vi "Frequency to phase word DBL.vi"(9 "Phase word base":i64=4294967296 format="0x%x (%d)", 10 "DDS clock":dbl=125000000.0 format="%_13p", 11 "Frequency":dbl format="%#_15p") -> (3 "Phase word":u64=1717987 format="0x%x (%d) 0b%b")   [LabVIEW 2015]
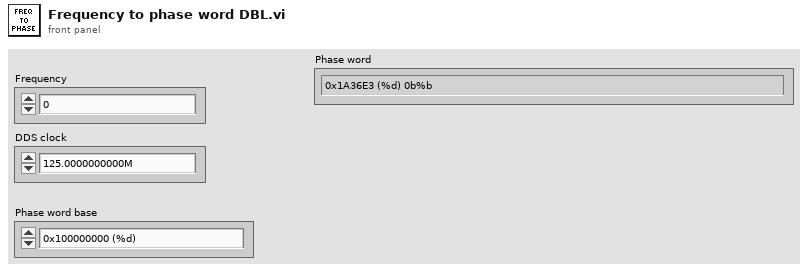
[diagram p1: front panel]
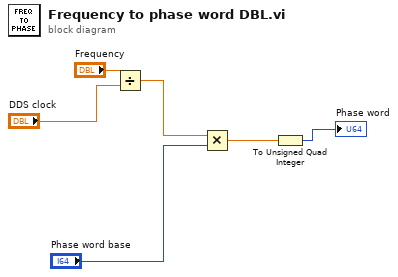
[diagram p0: block diagram]
diagram:
  n1 = Divide(x="Frequency", y="DDS clock") -> (x/y=w4:dbl)
  n2 = Multiply(x=w4, y="Phase word base") -> (x*y=w3:dbl)
  n3 = To Unsigned Quad Integer(1:w3) -> (0:→"Phase word":u64)
